vi "Fetch.vi"(8 "error in (no error)":errorcluster, 11 "VISA resource name":refnum<visa-resource-name>) -> (0 "error out":errorcluster, 1 "Secondary Measurement":dbl, 2 "Primary Measurement":dbl, 3 "VISA resource name out":refnum<visa-resource-name>)   [LabVIEW 2020, in "BK Precision 5491B.lvlib"]
doc: "Fetches a single measurement of the primary and secondary functions from the instrument.\n\n<b>Note: In order to read measurements of the secondary function, the secondary display must first be enabled using Enable Secondary Display.vi.</b>"
uses:
  <instrlib>/BK Precision 5491B/BK Precision 5491B.lvlib
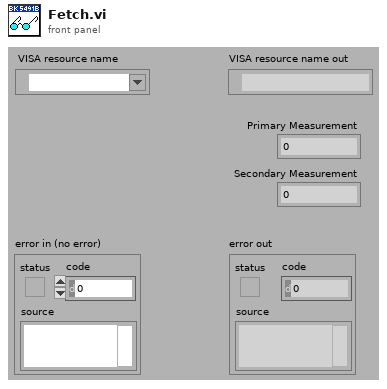
[diagram p1: front panel]
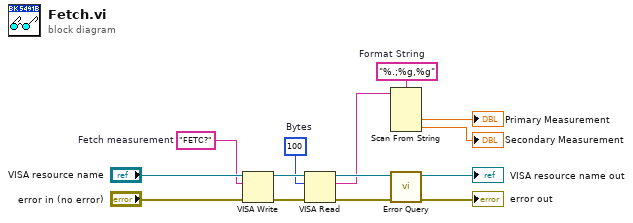
[diagram p0: block diagram]
diagram:
  w1 = "FETC?"  # Fetch measurement
  w6 = "%.;%g,%g"  # Format String
  w12 = u32 100  # Bytes
  n1 = VISA Write(VISA resource name="VISA resource name", write buffer=w1, error in (no error)="error in (no error)") -> (VISA resource name out=w13:refnum<visa-resource-name>, error out=w14:errorcluster)  [unwired: 1 out]
  n2 = VISA Read(VISA resource name=w13, byte count=w12, error in (no error)=w14) -> (VISA resource name out=w11:refnum<visa-resource-name>, read buffer=w7:string, error out=w10:errorcluster)  [unwired: 1 out]
  n3 = Scan From String(format string=w6, input string=w7) -> (output 1=→"Primary Measurement":dbl, output 2=→"Secondary Measurement":dbl)  [unwired: 4 in, 3 out]
  n4 = call <instrlib>:"Error Query.vi"("error in (no error)"=w10, "VISA resource name"=w11) -> ("error out"=→"error out":errorcluster, "VISA resource name out"=→"VISA resource name out":refnum<visa-resource-name>)  [unwired: 7 in, 1 out]
